vi "He4 Mano Read.vi"(2 "Range":enum16{"X 1", "X 0.1", "X 0.01", "X 0.001"}(ring), 3 "GPIB Address":string="08") -> (0 "Temperature (K)":dbl=1.5186540261408754 format="%.2f", 1 "Vapor pressure (torr)":dbl=3.8689999999999998 format="%.4f")   [LabVIEW 2009]
doc: "Reads the He4 vapor pressure and converts to a temperature."
panel:
  # "Electronic Manometer"
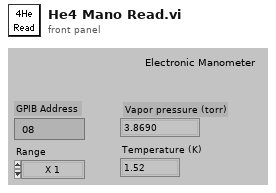
[diagram p1: front panel]
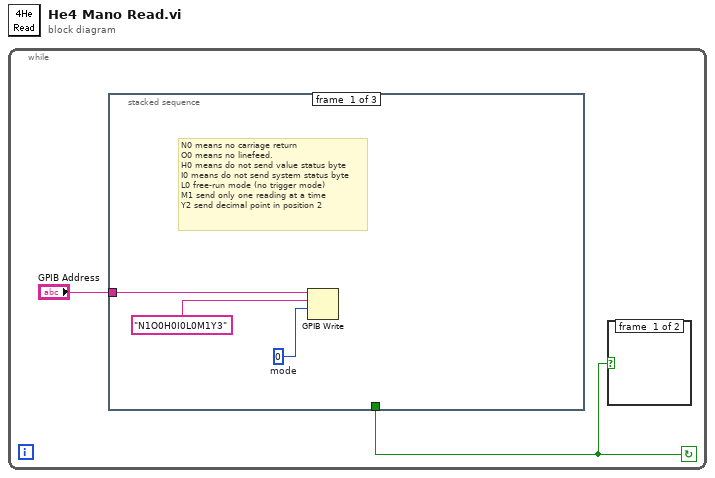
[diagram p0: block diagram]
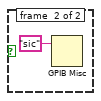
[diagram p2: hidden frame]
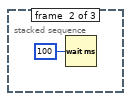
[diagram p3: hidden frame]
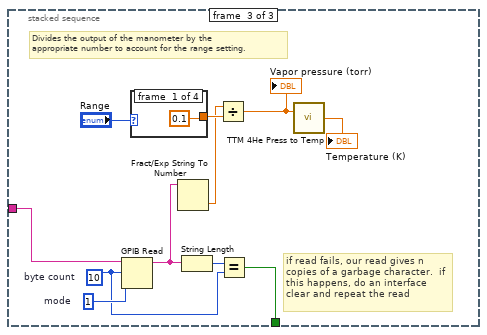
[diagram p4: hidden frame]
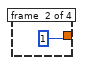
[diagram p5: hidden frame]
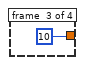
[diagram p6: hidden frame]
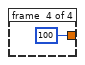
[diagram p7: hidden frame]
diagram:
  n1 = while {
    stop <- w1 continue-if-true
    n2 = stacked-sequence {
      tunnel: "GPIB Address" -> [w4 _ w17]
      tunnel: [_ _ w8] -> w1
      frame #0 {
        w6 = 0  # mode
        # "N0 means no carriage return\nO0 means no linefeed.\nH0 means do not send value status byte\nI0 means do not send system status byte\nL0 free-run mode (no trigger mode)\nM1 send only one reading at a time\nY2 send decimal point in position 2"
        n3 = GPIB Write(0:w4, 1:"N1O0H0I0L0M1Y3", 2:w6) -> ()  [unwired: 2 in, 2 out]
      }
      frame #1 {
        n4 = Wait (ms)(milliseconds to wait=u32 100) -> ()  [unwired: 1 out]
      }
      frame #2 {
        w9 = 10  # byte count
        w18 = 1  # mode
        # "if read fails, our read gives n copies of a garbage character.  if this happens, do an interface clear and repeat the read"
        # "Divides the output of the manometer by the\nappropriate number to account for the range setting."
        n5 = GPIB Read(0:w17, 1:w9, 2:w18) -> (5:w11:string)  [unwired: 2 in, 2 out]
        n6 = case shown="\"X 1\"" "Range" {
          tunnel: [0.1 1 10 100] -> w15
          frame #0 {
          }
          frame #1 {
          }
          frame #2 {
          }
          frame #3 {
          }
        }
        n7 = Fract/Exp String To Number(string=w11) -> (number=w14:dbl)  [unwired: 3 in, 1 out]
        n8 = String Length(string=w11) -> (length=w10:i32)
        n9 = Divide(x=w14, y=w15) -> (x/y=w12:dbl)
        "Vapor pressure (torr)" <- w12
        n10 = Equal?(x=w10, y=w9) -> (x = y?=w8:bool)
        n11 = call "TTM 4He Press to Temp.vi"("4He Vapor Pressure (torr)"=w12) -> ("4He Temp (K)"=→"Temperature (K)":dbl)
      }
    }
    n12 = case shown="True" w1 {
      frame #0 {
      }
      frame #1 {
        n13 = GPIB Misc(0:"sic" ("command string")) -> ()  [unwired: 1 in, 3 out]
      }
    }
  }
